vi "FIR&IIR+FFT_subVI.vi"(0 "waveform array IN":waveform(dbl)[](array[waveform]), 3 "optional FIR filter specifications":T3={"PB Gain"=-3.0, "SB Gain"=-60.0, "Scale"=TRUE, "Window"=enum."Flat Top"} {"SB Gain" format="%.2p"; "PB Gain" format="%.2p"}, 7 "error in (no error)":errorcluster, 9 "FIR / IIR":bool, 10 "FIR filter specifications":T4={"Topology"=enum."Off", "Type"=enum."Lowpass", "#Taps"=50, "Lower PB"=100.0, "Upper PB"=0.0, "Lower SB"=200.0, "Upper SB"=0.0} {"Lower SB" format="%0.2p"; "Upper SB" format="%0.2p"; "Lower PB" format="%0.2p"; "Upper PB" format="%0.2p"}, 11 "db ON":bool, 13 "optional IIR filter specifications":T1={"Lower PB"=100.0, "Upper PB"=0.0, "Lower SB"=200.0, "Upper SB"=0.0, "PB Gain"=-3.0, "SB Gain"=-60.0, "Scale"=TRUE} {"PB Gain" format="%0.2f"; "SB Gain" format="%0.2f"; "Lower SB" format="%0.2p"; "Upper SB" format="%0.2f"; "Lower PB" format="%0.2p"; "Upper PB" format="%0.2f"}, 14 "IIR filter specifications":T2={"Topology"=enum."Butterworth", "Type"=enum."Lowpass", "Order"=1, "Lower Fc"=100.0, "Upper Fc"=200.0, "PB Ripple"=1.0, "SB Attenuation"=60.0} {"PB Ripple" format="%0.2f"; "SB Attenuation" format="%0.2f"; "Lower Fc" format="%0.2p"; "Upper Fc" format="%0.2p"}) -> (1 "magnitude":cluster{"f0":dbl, "df":dbl, "magnitude":dbl[]} {"magnitude" format="%.2p"; "f0" format="%0.2p"; "df" format="%0.2p"}, 4 "t0":timestamp, 5 "FIR ON":bool, 6 "Signal":waveform(dbl)[](array[waveform]), 8 "error out":errorcluster, 15 "IIR ON":bool)   [LabVIEW 2018]
uses:
  <vilib>/Waveform/WDTOps.llb/WDT Index Channel DBL.vi
  <vilib>/measure/macond.llb/IIR Filter for 1 Chan.vi
  <vilib>/measure/macond.llb/FIR Filter for 1 Chan.vi
  <vilib>/measure/maspectr.llb/FFT Spectrum (Mag-Phase) for 1 Chan.vi
  <vilib>/measure/NI_MAPro.lvlib
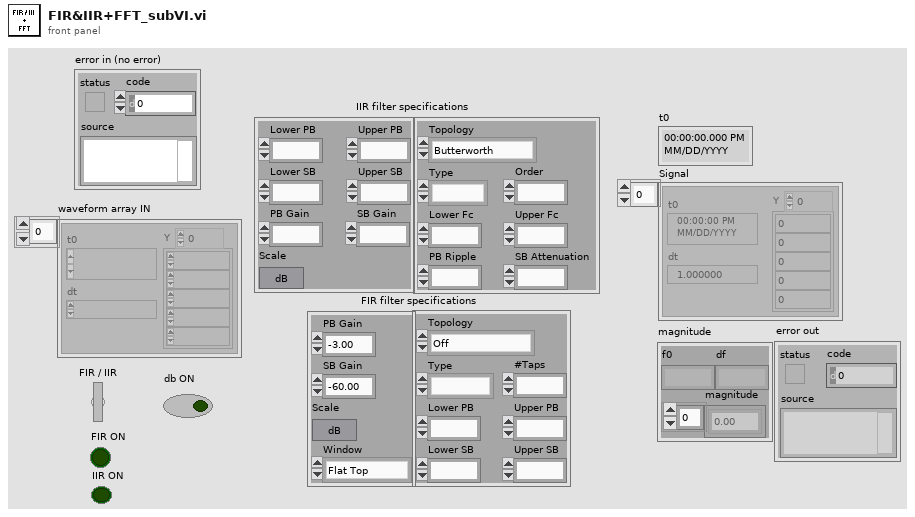
[diagram p1: front panel]
types:
  T1 = cluster{"Lower PB":dbl, "Upper PB":dbl, "Lower SB":dbl, "Upper SB":dbl, "PB Gain":dbl, "SB Gain":dbl, "Scale":bool}
  T2 = cluster{"Topology":enum16{"Off", "Butterworth", "Chebyshev", "Inverse Chebyshev", "Elliptic", "Bessel"}, "Type":enum16{"Lowpass", "Highpass", "Bandpass", "Bandstop"}, "Order":i32, "Lower Fc":dbl, "Upper Fc":dbl, "PB Ripple":dbl, "SB Attenuation":dbl}
  T3 = cluster{"PB Gain":dbl, "SB Gain":dbl, "Scale":bool, "Window":enum16{"None", "Hanning", "Hamming", "Triangular", "Blackman", "Exact Blackman", "Blackman-Harris", "Kaiser-Bessel", "Flat Top"}}
  T4 = cluster{"Topology":enum16{"Off", "FIR by Specification", "Equi-ripple FIR", "Windowed FIR"}, "Type":enum16{"Lowpass", "Highpass", "Bandpass", "Bandstop"}, "#Taps":i32, "Lower PB":dbl, "Upper PB":dbl, "Lower SB":dbl, "Upper SB":dbl}
  T5 = cluster{"dB On (F)":bool, "unwrap phase (F)":bool, "convert to degree (F)":bool}
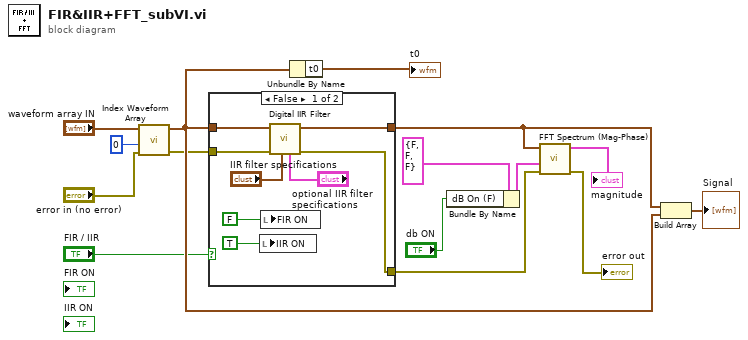
[diagram p0: block diagram]
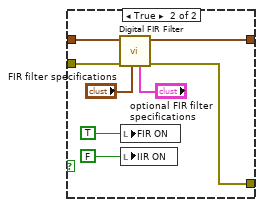
[diagram p2: hidden frame]
diagram:
  n1 = call-poly <vilib>:"Index Waveform Array.vi"("error in (no error)"="error in (no error)", "index"=0, "waveform array"="waveform array IN") -> ("error out"=w2:errorcluster, "waveform"=w11:waveform(dbl))  [unwired: 7 in]
  n2 = case shown="False" "FIR / IIR" {
    tunnel: w11 -> [w23 w29]
    tunnel: [w20 w28] -> w10
    tunnel: [w17 w25] -> w5
    tunnel: w2 -> [w16 w24]
    frame False {
      n3 = local write "IIR ON"(TRUE ("IIR ON")) -> ()
      n4 = local write "FIR ON"(FALSE ("FIR ON")) -> ()
      n5 = call-poly <vilib>:"Digital IIR Filter.vi"("optional IIR filter specifications"="optional IIR filter specifications", "IIR filter specifications"="IIR filter specifications", "error in (no error)"=w16, "signal in"=w23) -> ("error out"=w17:errorcluster, "signal out"=w20:waveform(dbl))  [unwired: 5 in, 1 out]
    }
    frame True {
      n6 = call-poly <vilib>:"Digital FIR Filter.vi"("optional FIR filter specifications"="optional FIR filter specifications", "FIR filter specifications"="FIR filter specifications", "error in (no error)"=w24, "signal in"=w29) -> ("error out"=w25:errorcluster, "signal out"=w28:waveform(dbl))  [unwired: 5 in, 1 out]
      n7 = local write "FIR ON"(TRUE ("FIR ON")) -> ()
      n8 = local write "IIR ON"(FALSE ("IIR ON")) -> ()
    }
  }
  n9 = Unbundle By Name(w11) -> ("t0"=→"t0":timestamp)
  n10 = Bundle By Name(cluster=T5 {"dB On (F)"=FALSE, "unwrap phase (F)"=FALSE, "convert to degree (F)"=FALSE} ("view"), "dB On (F)"="db ON") -> (w13:T5)
  n11 = call-poly <vilib>:"FFT Spectrum (Mag-Phase).vi"("error in (no error)"=w5, "view"=w13, "time signal"=w10) -> ("error out"=→"error out":errorcluster, "magnitude"=→"magnitude":cluster{"f0":dbl, "df":dbl, "magnitude":dbl[]})  [unwired: 4 in, 3 out]
  n12 = Build Array(w10, w11) -> (→"Signal":waveform(dbl)[])
